vi "Convert To Absolute Path.vi"(1 "System Definition File Path":path) -> (0 "Absolute path":path)   [LabVIEW 2019, in "TLCD Test Class.lvclass"]
uses:
  TLCD Test Class.lvclass
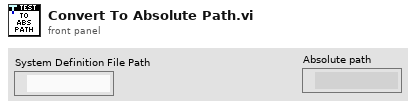
[diagram p1: front panel]
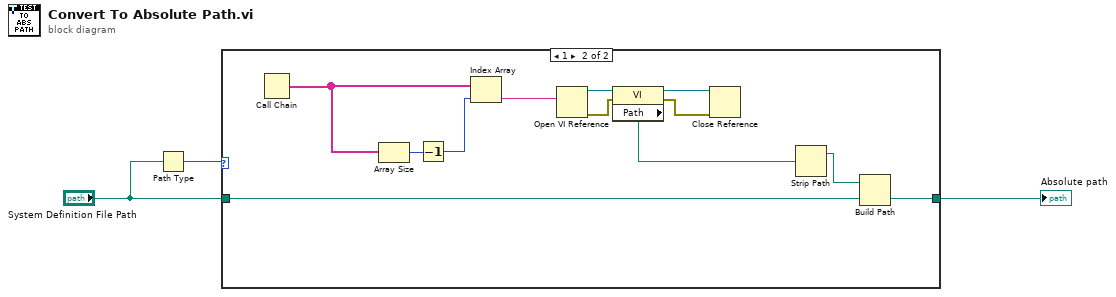
[diagram p0: block diagram]
diagram:
  n1 = Path Type(1:"System Definition File Path") -> (0:w1:i16)
  n2 = case shown="1" w1 {
    tunnel: [w4 w6] -> w3
    tunnel: "System Definition File Path" -> [w4 w5]
    frame 0, Default {
    }
    frame 1 {
      n3 = Call Chain() -> (call chain=w15:string[])
      n4 = Array Size(array=w15) -> (size(s)=w16:i32)
      n5 = Decrement(x=w16) -> (x-1=w14:i32)
      n6 = Index Array(array=w15, index=w14) -> (element=w13:string)
      n7 = Open VI Reference(vi path=w13) -> (vi reference=w12:refnum<vi>, error out=w11:errorcluster)  [unwired: 5 in]
      n8 = property class="VI"(reference=w12, error in=w11) -> (reference out=w9:refnum<vi>, error out=w10:errorcluster, "Path"=w8:path)
      n9 = Close Reference(reference=w9, error in (no error)=w10) -> ()  [unwired: 1 out]
      n10 = Strip Path(path=w8) -> (stripped path=w7:path)  [unwired: 1 out]
      n11 = Build Path(base path=w7, name or relative path=w5) -> (appended path=w6:path)
    }
  }
  "Absolute path" <- w3
